vi "BkgGradient.vi"(11 "General settings":T1) -> (0 "Holo mask":dbl[][](array[numeric]), 3 "gradient":dbl[][](array[numeric]))   [LabVIEW 2018]
uses:
  Controls/General Setting.ctl
  Controls/Buttons/Running Button.ctl
panel:
  out "Gradient Graph":dbl[][](graph)
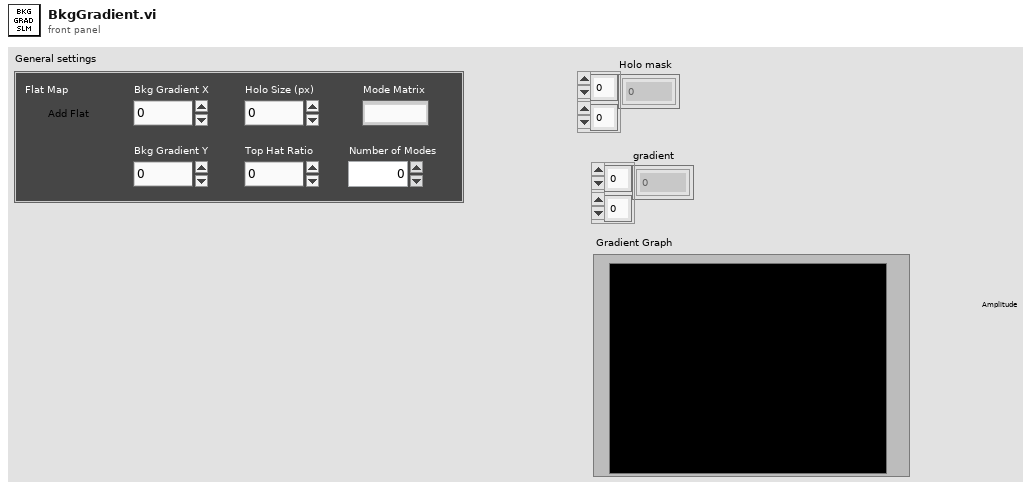
[diagram p1: front panel]
types:
  T1 = typedef "General Setting.ctl" = cluster{"Flat Map":T2, "Bkg Gradient X":dbl, "Bkg Gradient Y":dbl, "Holo Size (px)":i32, "Top Hat Ratio":dbl, "Number of Modes":i8, "Mode Matrix":u16}
  T2 = typedef "Running Button.ctl" = bool
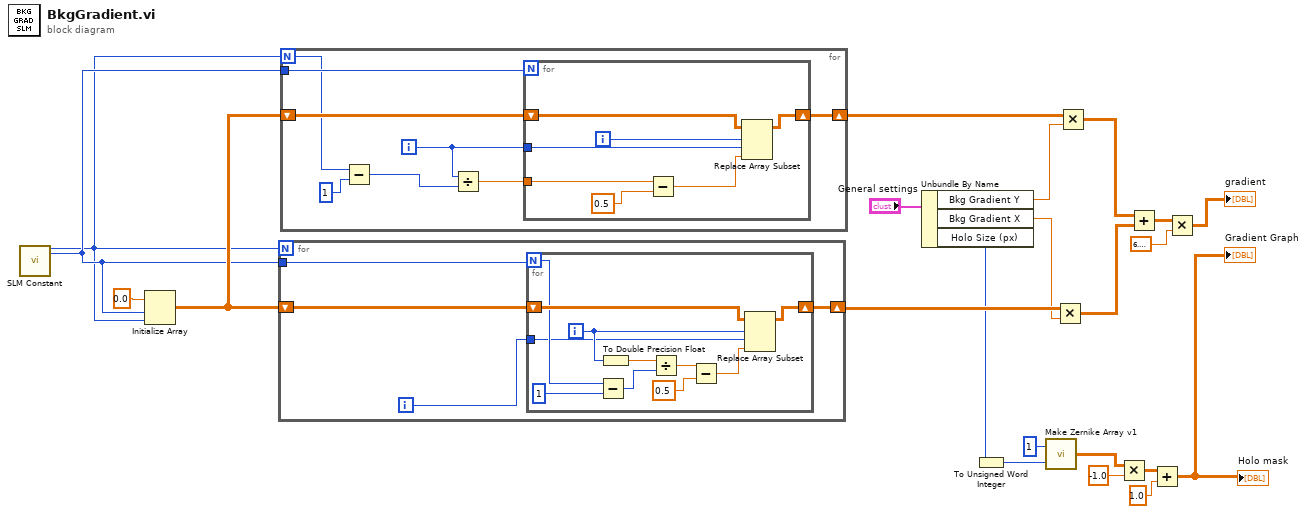
[diagram p0: block diagram]
diagram:
  n1 = call "SLM Constant.vi"() -> ("Lateral Effective Pixel Number"=w6:i32, "Vertical (Effective) Pixel Number"=w7:i32)  [unwired: 10 in, 8 out]
  n2 = Initialize Array(0.0 ("element"), w7, w6) -> (w22:dbl[][])
  n3 = for {
    N: w6 -> [_]
    tunnel: w7 -> [w25]
    shift-right: [w24] -> w14
    shift-left: w22 -> [w26]
    i -> [w23]
    n4 = for {
      N: w25 -> [w29]
      shift-right: [w36] -> w24
      shift-left: w26 -> [w35]
      tunnel: w23 -> [w27]
      i -> [w37]
      n5 = Subtract(x=w29, y=1) -> (x-y=w30:i32)
      n6 = To Double Precision Float(number=w37) -> (double precision float=w34:dbl)
      n7 = Divide(x=w34, y=w30) -> (x/y=w32:dbl)
      n8 = Subtract(x=w32, y=0.5 ("element")) -> (x-y=w31:dbl)
      n9 = Replace Array Subset(array=w35, new element=w31, index (row)=w37, index (col)=w27) -> (w36:dbl[][])
    }
  }
  n10 = for {
    N: w6 -> [w39]
    tunnel: w7 -> [w44]
    shift-right: [w43] -> w15
    shift-left: w22 -> [w45]
    i -> [w42]
    n11 = Subtract(x=w39, y=1) -> (x-y=w38:i32)
    n12 = Divide(x=w42, y=w38) -> (x/y=w41:dbl)
    n13 = for {
      N: w44 -> [_]
      shift-right: [w51] -> w43
      shift-left: w45 -> [w50]
      tunnel: w42 -> [w49]
      tunnel: w41 -> [w48]
      i -> [w52]
      n14 = Subtract(x=w48, y=0.5) -> (x-y=w47:dbl)
      n15 = Replace Array Subset(array=w50, new element=w47, index (row)=w52, index (col)=w49) -> (w51:dbl[][])
    }
  }
  n16 = Unbundle By Name("General settings") -> ("Bkg Gradient Y"=w11:dbl, "Bkg Gradient X"=w10:dbl, "Holo Size (px)"=w9:i32)
  n17 = To Unsigned Word Integer(number=w9) -> (unsigned 16bit integer=w8:u16)
  n18 = call "Make Zernike Array v1.vi"("size"=w8, "z"=u8 1) -> ("zernike array"=w18:dbl[][])
  n19 = Multiply(x=w14, y=w10) -> (x*y=w5:dbl[][])
  n20 = Multiply(x=w15, y=w11) -> (x*y=w13:dbl[][])
  n21 = Multiply(x=w18, y=-1.0) -> (x*y=w17:dbl[][])
  n22 = Add(x=w13, y=w5) -> (x+y=w4:dbl[][])
  n23 = Add(x=w17, y=1.0) -> (x+y=→"Holo mask" →"Gradient Graph":dbl[][])
  n24 = Multiply(x=w4, y=6.283185307179586) -> (x*y=→"gradient":dbl[][])
